vi "_StateStatus.vi"(0 "Device Name":string) -> (1 "Error Code":i32, 2 "Error Stack":string[](array[string]), 3 "State Code":i16, 4 "State Color":u32(colorbox)=16448250, 5 "State String":string, 6 "Status":string)   [LabVIEW 2014, in "tango.lvlib"]
uses:
  tango.lvlib
  tango_binding.so
panel:
  out "State/Status":string[](array[string])
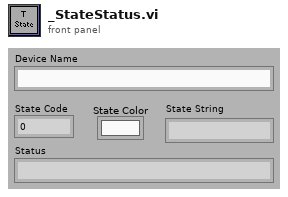
[diagram p1: front panel]
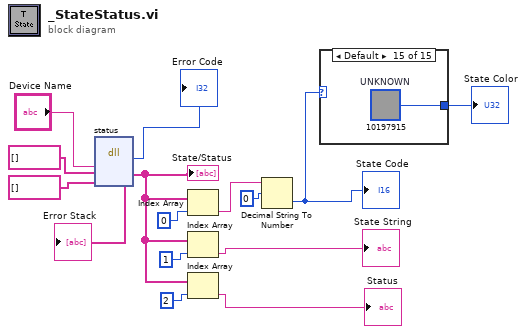
[diagram p0: block diagram]
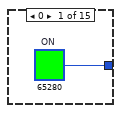
[diagram p2: hidden frame]
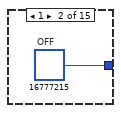
[diagram p3: hidden frame]
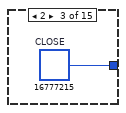
[diagram p4: hidden frame]
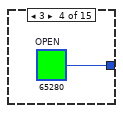
[diagram p5: hidden frame]
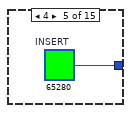
[diagram p6: hidden frame]
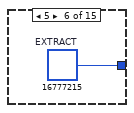
[diagram p7: hidden frame]
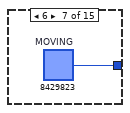
[diagram p8: hidden frame]
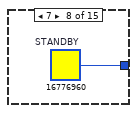
[diagram p9: hidden frame]
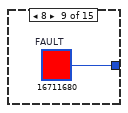
[diagram p10: hidden frame]
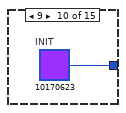
[diagram p11: hidden frame]
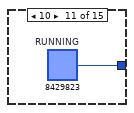
[diagram p12: hidden frame]
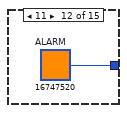
[diagram p13: hidden frame]
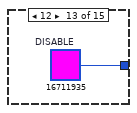
[diagram p14: hidden frame]
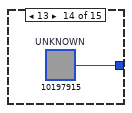
[diagram p15: hidden frame]
diagram:
  n1 = dll-call lib="tango_binding.*" fn="status"("dev_name"="Device Name", "status"=string[] [] ("State/Status"), "error_stack"=string[] [] ("Error Stack")) -> (→"Error Code":i32, "status"=w10:string[], "error_stack"=→"Error Stack":string[])  [unwired: 4 in, 2 out]
  "State/Status" <- w10
  n2 = Index Array(array=w10, index=0 ("indice")) -> (element=w9:string)
  n3 = Index Array(array=w10, index=1 ("indice")) -> (element=→"State String":string)
  n4 = Index Array(array=w10, index=2 ("indice")) -> (element=→"Status":string)
  n5 = Decimal String To Number(string=w9, offset=0) -> (number=w3:i32)  [unwired: 1 in, 1 out]
  "State Code" <- w3
  n6 = case shown="Default" w3 {
    tunnel: [w16 w17 w18 w19 w20 w21 w22 w23 w24 w25 w26 w27 w28 w29 w30] -> w5
    frame 0 {
      w16 = u32 65280  # ON
    }
    frame 1 {
      w17 = u32 16777215  # OFF
    }
    frame 2 {
      w18 = u32 16777215  # CLOSE
    }
    frame 3 {
      w19 = u32 65280  # OPEN
    }
    frame 4 {
      w20 = u32 65280  # INSERT
    }
    frame 5 {
      w21 = u32 16777215  # EXTRACT
    }
    frame 6 {
      w22 = u32 8429823  # MOVING
    }
    frame 7 {
      w23 = u32 16776960  # STANDBY
    }
    frame 8 {
      w24 = u32 16711680  # FAULT
    }
    frame 9 {
      w25 = u32 10170623  # INIT
    }
    frame 10 {
      w26 = u32 8429823  # RUNNING
    }
    frame 11 {
      w27 = u32 16747520  # ALARM
    }
    frame 12 {
      w28 = u32 16711935  # DISABLE
    }
    frame 13 {
      w29 = u32 10197915  # UNKNOWN
    }
    frame Default {
      w30 = u32 10197915  # UNKNOWN
    }
  }
  "State Color" <- w5
